vi "Hatch.vi"(10 "Polys":T4[](array[typedef]), 11 "Hatch":T4) -> (3 "Path":T2)   [LabVIEW 2014]
uses:
  TypeDefs/Poly2D.ctl
  TypeDefs/Point2D.ctl
panel:
  out "XY Graph":T3(graph)
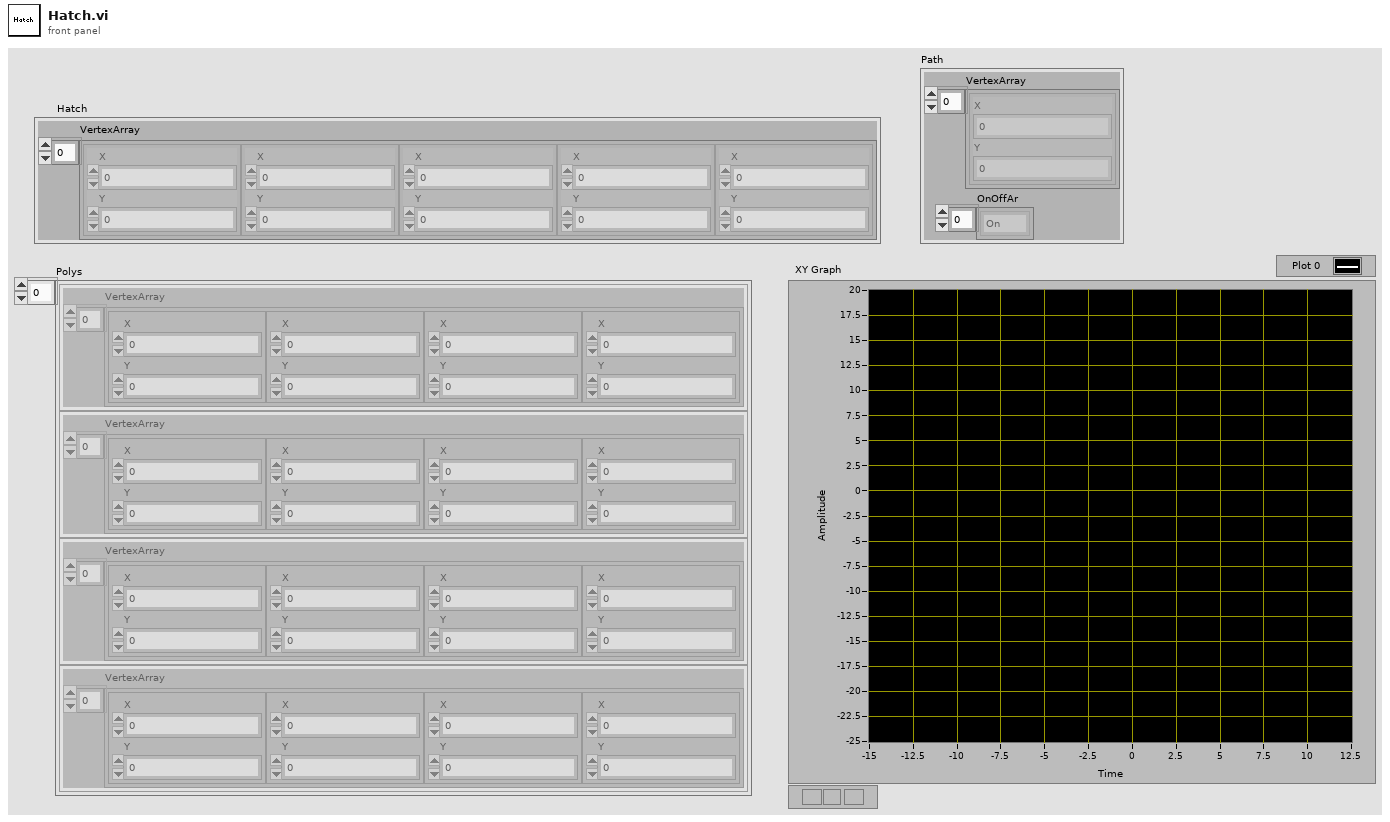
[diagram p1: front panel]
types:
  T1 = typedef "Point2D.ctl" = cluster{"X":sgl, "Y":sgl}
  T2 = cluster{"VertexArray":T1[], "OnOffAr":enum16{"On", "Off"}[]}
  T3 = cluster{"VertexArray":cluster{"X":sgl, "Y":sgl}[]}[]
  T4 = typedef "Poly2D.ctl" = cluster{"VertexArray":T1[]}
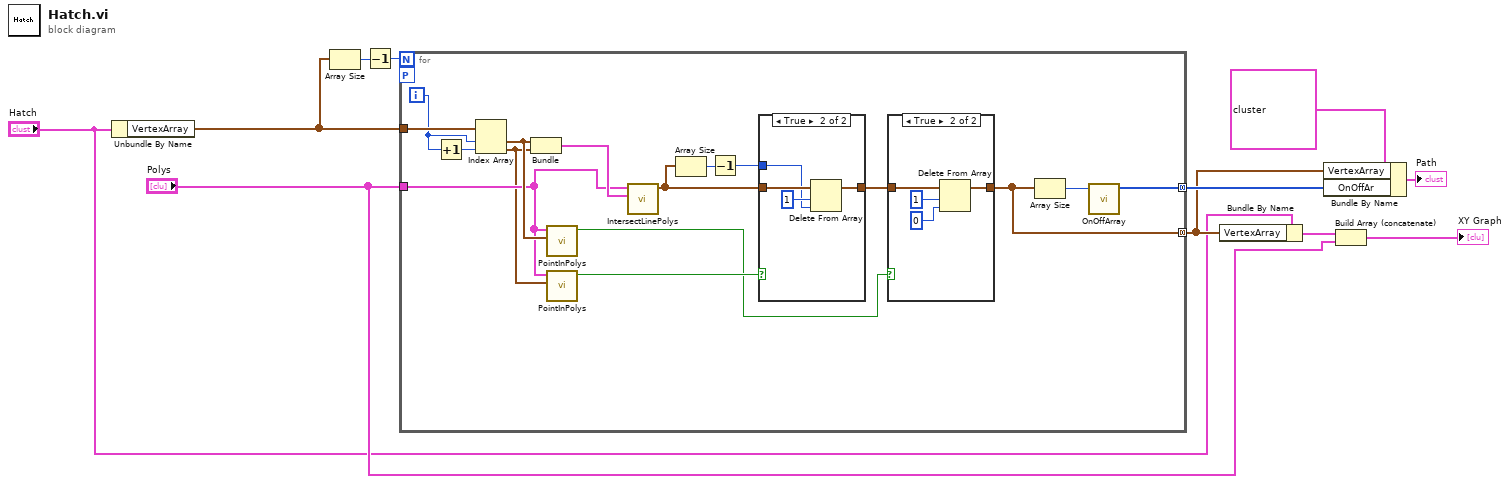
[diagram p0: block diagram]
diagram:
  n1 = Unbundle By Name("Hatch") -> ("VertexArray"=w1:T1[])
  n2 = Array Size(array=w1) -> (size(s)=w11:i32)
  n3 = Decrement(x=w11) -> (x-1=w10:i32)
  n4 = for {
    N: w10 -> [_]
    tunnel: w1 -> [w27]
    tunnel: "Polys" -> [w22]
    tunnel: [w13] -> w5 mode=concatenating
    tunnel: [w12] -> w4 mode=concatenating
    workers-P: _ -> [_]
    i -> [w25]
    n5 = Increment(x=w25) -> (x+1=w26:i32)
    n6 = Index Array(array=w27, index #1=w25, index #2=w26) -> (element #1=w24:T1, element #2=w21:T1)
    n7 = Bundle("Point2D"=w24, "Point2D"=w21) -> (w23:cluster{"Point2D":T1, "Point2D":T1})  [unwired: 1 in]
    n8 = call "PointInPolys.vi"("Point2D"=w24, "Polys"=w22) -> ("Outside"=w15:bool)  [unwired: 9 in]
    n9 = call "PointInPolys.vi"("Point2D"=w21, "Polys"=w22) -> ("Outside"=w19:bool)  [unwired: 9 in]
    n10 = call "IntersectLinePolys.vi"("Line2D"=w23, "Polys"=w22) -> ("Intersections"=w18:T1[])  [unwired: 9 in]
    n11 = Array Size(array=w18) -> (size(s)=w20:i32)
    n12 = Decrement(x=w20) -> (x-1=w17:i32)
    n13 = case shown="True" w19 {
      tunnel: w18 -> [w33 w37]
      tunnel: w17 -> [_ w35]
      tunnel: [w33 w34] -> w16
      frame False {
      }
      frame True {
        n14 = Delete From Array(array=w37, length=1, index=w35) -> (array with subset deleted=w34:T1[])  [unwired: 1 out]
      }
    }
    n15 = case shown="True" w15 {
      tunnel: w16 -> [w28 w32]
      tunnel: [w28 w30] -> w12
      frame False {
      }
      frame True {
        n16 = Delete From Array(array=w32, length=1, index=0) -> (array with subset deleted=w30:T1[])  [unwired: 1 out]
      }
    }
    n17 = Array Size(array=w12) -> (size(s)=w14:i32)
    n18 = call "OnOffArray.vi"("Size"=w14) -> ("OnOffAr"=w13:enum16{"On", "Off"}[])  [unwired: 10 in]
  }
  n19 = Bundle By Name(cluster="Hatch", "VertexArray"=w4) -> (w9:T4)
  n20 = Bundle By Name(cluster=T2 {"VertexArray"=[{"X"=-16.0, "Y"=-26.0}, {"X"=12.0, "Y"=-26.0}, {"X"=12.0, "Y"=-25.9}, {"X"=-16.0, "Y"=-25.9}, {"X"=-16.0, "Y"=-25.8}, {"X"=12.0, "Y"=-25.8}, {"X"=12.0, "Y"=-25.7}, {"X"=-16.0, "Y"=-25.7}, {"X"=-16.0, "Y"=-25.6}, {"X"=12.0, "Y"=-25.6}, {"X"=12.0, "Y"=-25.5}, {"X"=-16.0, "Y"=-25.5}, {"X"=-16.0, "Y"=-25.4}, {"X"=12.0, "Y"=-25.4}, {"X"=12.0, "Y"=-25.3}, {"X"=-16.0, "Y"=-25.3}, {"X"=-16.0, "Y"=-25.2}, {"X"=12.0, "Y"=-25.2}, {"X"=12.0, "Y"=-25.1}, {"X"=-16.0, "Y"=-25.1}, {"X"=-16.0, "Y"=-25.0}, {"X"=12.0, "Y"=-25.0}, {"X"=12.0, "Y"=-24.9}, {"X"=-16.0, "Y"=-24.9}, {"X"=-16.0, "Y"=-24.8}, {"X"=12.0, "Y"=-24.8}, {"X"=12.0, "Y"=-24.7}, {"X"=-16.0, "Y"=-24.7}, {"X"=-16.0, "Y"=-24.6}, {"X"=12.0, "Y"=-24.6}, {"X"=12.0, "Y"=-24.5}, {"X"=-16.0, "Y"=-24.5}, {"X"=-16.0, "Y"=-24.4}, {"X"=12.0, "Y"=-24.4}, {"X"=12.0, "Y"=-24.3}, {"X"=-16.0, "Y"=-24.3}, {"X"=-16.0, "Y"=-24.2}, {"X"=12.0, "Y"=-24.2}, {"X"=12.0, "Y"=-24.1}, {"X"=-16.0, "Y"=-24.1}, {"X"=-16.0, "Y"=-24.0}, {"X"=12.0, "Y"=-24.0}, {"X"=12.0, "Y"=-23.9}, {"X"=-16.0, "Y"=-23.9}, {"X"=-16.0, "Y"=-23.8}, {"X"=12.0, "Y"=-23.8}, {"X"=12.0, "Y"=-23.7}, {"X"=-16.0, "Y"=-23.7}, {"X"=-16.0, "Y"=-23.6}, {"X"=12.0, "Y"=-23.6}, {"X"=12.0, "Y"=-23.5}, {"X"=-16.0, "Y"=-23.5}, {"X"=-16.0, "Y"=-23.4}, {"X"=12.0, "Y"=-23.4}, {"X"=12.0, "Y"=-23.3}, {"X"=-16.0, "Y"=-23.3}, {"X"=-16.0, "Y"=-23.2}, {"X"=12.0, "Y"=-23.2}, {"X"=12.0, "Y"=-23.1}, {"X"=-16.0, "Y"=-23.1}, {"X"=-16.0, "Y"=-23.0}, {"X"=12.0, "Y"=-23.0}, {"X"=12.0, "Y"=-22.9}, {"X"=-16.0, "Y"=-22.9}, {"X"=-16.0, "Y"=-22.8}, {"X"=12.0, "Y"=-22.8}, {"X"=12.0, "Y"=-22.7}, {"X"=-16.0, "Y"=-22.7}, {"X"=-16.0, "Y"=-22.6}, {"X"=12.0, "Y"=-22.6}, {"X"=12.0, "Y"=-22.5}, {"X"=-16.0, "Y"=-22.5}, {"X"=-16.0, "Y"=-22.4}, {"X"=12.0, "Y"=-22.4}, {"X"=12.0, "Y"=-22.3}, {"X"=-16.0, "Y"=-22.3}, {"X"=-16.0, "Y"=-22.2}, {"X"=12.0, "Y"=-22.2}, {"X"=12.0, "Y"=-22.1}, {"X"=-16.0, "Y"=-22.1}, {"X"=-16.0, "Y"=-22.0}, {"X"=12.0, "Y"=-22.0}, {"X"=12.0, "Y"=-21.9}, {"X"=-16.0, "Y"=-21.9}, {"X"=-16.0, "Y"=-21.8}, {"X"=12.0, "Y"=-21.8}, {"X"=12.0, "Y"=-21.7}, {"X"=-16.0, "Y"=-21.7}, {"X"=-16.0, "Y"=-21.6}, {"X"=12.0, "Y"=-21.6}, {"X"=12.0, "Y"=-21.5}, {"X"=-16.0, "Y"=-21.5}, {"X"=-16.0, "Y"=-21.4}, {"X"=12.0, "Y"=-21.4}, {"X"=12.0, "Y"=-21.3}, {"X"=-16.0, "Y"=-21.3}, {"X"=-16.0, "Y"=-21.2}, {"X"=12.0, "Y"=-21.2}, {"X"=12.0, "Y"=-21.1}, {"X"=-16.0, "Y"=-21.1}, {"X"=-16.0, "Y"=-21.0}, {"X"=12.0, "Y"=-21.0}, {"X"=12.0, "Y"=-20.9}, {"X"=-16.0, "Y"=-20.9}, {"X"=-16.0, "Y"=-20.8}, {"X"=12.0, "Y"=-20.8}, {"X"=12.0, "Y"=-20.7}, {"X"=-16.0, "Y"=-20.7}, {"X"=-16.0, "Y"=-20.6}, {"X"=12.0, "Y"=-20.6}, {"X"=12.0, "Y"=-20.5}, {"X"=-16.0, "Y"=-20.5}, {"X"=-16.0, "Y"=-20.4}, {"X"=12.0, "Y"=-20.4}, {"X"=12.0, "Y"=-20.3}, {"X"=-16.0, "Y"=-20.3}, {"X"=-16.0, "Y"=-20.2}, {"X"=12.0, "Y"=-20.2}, {"X"=12.0, "Y"=-20.1}, {"X"=-16.0, "Y"=-20.1}, {"X"=-16.0, "Y"=-20.0}, {"X"=12.0, "Y"=-20.0}, {"X"=12.0, "Y"=-19.9}, {"X"=-16.0, "Y"=-19.9}, {"X"=-16.0, "Y"=-19.8}, {"X"=12.0, "Y"=-19.8}, {"X"=12.0, "Y"=-19.7}, {"X"=-16.0, "Y"=-19.7}, {"X"=-16.0, "Y"=-19.6}, {"X"=12.0, "Y"=-19.6}, {"X"=12.0, "Y"=-19.5}, {"X"=-16.0, "Y"=-19.5}, {"X"=-16.0, "Y"=-19.4}, {"X"=12.0, "Y"=-19.4}, {"X"=12.0, "Y"=-19.3}, {"X"=-16.0, "Y"=-19.3}, {"X"=-16.0, "Y"=-19.2}, {"X"=12.0, "Y"=-19.2}, {"X"=12.0, "Y"=-19.1}, {"X"=-16.0, "Y"=-19.1}, {"X"=-16.0, "Y"=-19.0}, {"X"=12.0, "Y"=-19.0}, {"X"=12.0, "Y"=-18.9}, {"X"=-16.0, "Y"=-18.9}, {"X"=-16.0, "Y"=-18.8}, {"X"=12.0, "Y"=-18.8}, {"X"=12.0, "Y"=-18.7}, {"X"=-16.0, "Y"=-18.7}, {"X"=-16.0, "Y"=-18.6}, {"X"=12.0, "Y"=-18.6}, {"X"=12.0, "Y"=-18.5}, {"X"=-16.0, "Y"=-18.5}, {"X"=-16.0, "Y"=-18.4}, {"X"=12.0, "Y"=-18.4}, {"X"=12.0, "Y"=-18.3}, {"X"=-16.0, "Y"=-18.3}, {"X"=-16.0, "Y"=-18.2}, {"X"=12.0, "Y"=-18.2}, {"X"=12.0, "Y"=-18.1}, {"X"=-16.0, "Y"=-18.1}, {"X"=-16.0, "Y"=-18.0}, {"X"=12.0, "Y"=-18.0}, {"X"=12.0, "Y"=-17.9}, {"X"=-16.0, "Y"=-17.9}, {"X"=-16.0, "Y"=-17.8}, {"X"=12.0, "Y"=-17.8}, {"X"=12.0, "Y"=-17.7}, {"X"=-16.0, "Y"=-17.7}, {"X"=-16.0, "Y"=-17.6}, {"X"=12.0, "Y"=-17.6}, {"X"=12.0, "Y"=-17.5}, {"X"=-16.0, "Y"=-17.5}, {"X"=-16.0, "Y"=-17.4}, {"X"=12.0, "Y"=-17.4}, {"X"=12.0, "Y"=-17.3}, {"X"=-16.0, "Y"=-17.3}, {"X"=-16.0, "Y"=-17.2}, {"X"=12.0, "Y"=-17.2}, {"X"=12.0, "Y"=-17.1}, {"X"=-16.0, "Y"=-17.1}, {"X"=-16.0, "Y"=-17.0}, {"X"=12.0, "Y"=-17.0}, {"X"=12.0, "Y"=-16.9}, {"X"=-16.0, "Y"=-16.9}, {"X"=-16.0, "Y"=-16.8}, {"X"=12.0, "Y"=-16.8}, {"X"=12.0, "Y"=-16.7}, {"X"=-16.0, "Y"=-16.7}, {"X"=-16.0, "Y"=-16.6}, {"X"=12.0, "Y"=-16.6}, {"X"=12.0, "Y"=-16.5}, {"X"=-16.0, "Y"=-16.5}, {"X"=-16.0, "Y"=-16.4}, {"X"=12.0, "Y"=-16.4}, {"X"=12.0, "Y"=-16.3}, {"X"=-16.0, "Y"=-16.3}, {"X"=-16.0, "Y"=-16.2}, {"X"=12.0, "Y"=-16.2}, {"X"=12.0, "Y"=-16.1}, {"X"=-16.0, "Y"=-16.1}, {"X"=-16.0, "Y"=-16.0}, {"X"=12.0, "Y"=-16.0}, {"X"=12.0, "Y"=-15.9}, {"X"=-16.0, "Y"=-15.9}, {"X"=-16.0, "Y"=-15.8}, {"X"=12.0, "Y"=-15.8}, {"X"=12.0, "Y"=-15.7}, {"X"=-16.0, "Y"=-15.7}, {"X"=-16.0, "Y"=-15.6}, {"X"=12.0, "Y"=-15.6}, {"X"=12.0, "Y"=-15.5}, {"X"=-16.0, "Y"=-15.5}, {"X"=-16.0, "Y"=-15.4}, {"X"=12.0, "Y"=-15.4}, {"X"=12.0, "Y"=-15.3}, {"X"=-16.0, "Y"=-15.3}, {"X"=-16.0, "Y"=-15.2}, {"X"=12.0, "Y"=-15.2}, {"X"=12.0, "Y"=-15.1}, {"X"=-16.0, "Y"=-15.1}, {"X"=-16.0, "Y"=-15.0}, {"X"=12.0, "Y"=-15.0}, {"X"=12.0, "Y"=-14.9}, {"X"=-16.0, "Y"=-14.9}, {"X"=-16.0, "Y"=-14.8}, {"X"=12.0, "Y"=-14.8}, {"X"=12.0, "Y"=-14.7}, {"X"=-16.0, "Y"=-14.7}, {"X"=-16.0, "Y"=-14.6}, {"X"=12.0, "Y"=-14.6}, {"X"=12.0, "Y"=-14.5}, {"X"=-16.0, "Y"=-14.5}, {"X"=-16.0, "Y"=-14.4}, {"X"=12.0, "Y"=-14.4}, {"X"=12.0, "Y"=-14.3}, {"X"=-16.0, "Y"=-14.3}, {"X"=-16.0, "Y"=-14.2}, {"X"=12.0, "Y"=-14.2}, {"X"=12.0, "Y"=-14.1}, {"X"=-16.0, "Y"=-14.1}, {"X"=-16.0, "Y"=-14.0}, {"X"=12.0, "Y"=-14.0}, {"X"=12.0, "Y"=-13.9}, {"X"=-16.0, "Y"=-13.9}, {"X"=-16.0, "Y"=-13.8}, {"X"=12.0, "Y"=-13.8}, {"X"=12.0, "Y"=-13.7}, {"X"=-16.0, "Y"=-13.7}, {"X"=-16.0, "Y"=-13.6}, {"X"=12.0, "Y"=-13.6}, {"X"=12.0, "Y"=-13.5}, {"X"=-16.0, "Y"=-13.5}, {"X"=-16.0, "Y"=-13.4}, {"X"=12.0, "Y"=-13.4}, {"X"=12.0, "Y"=-13.3}, {"X"=-16.0, "Y"=-13.3}, {"X"=-16.0, "Y"=-13.2}, {"X"=12.0, "Y"=-13.2}, {"X"=12.0, "Y"=-13.1}, {"X"=-16.0, "Y"=-13.1}, {"X"=-16.0, "Y"=-13.0}, {"X"=12.0, "Y"=-13.0}, {"X"=12.0, "Y"=-12.9}, {"X"=-16.0, "Y"=-12.9}, {"X"=-16.0, "Y"=-12.8}, {"X"=12.0, "Y"=-12.8}, {"X"=12.0, "Y"=-12.7}, {"X"=-16.0, "Y"=-12.7}, {"X"=-16.0, "Y"=-12.6}, {"X"=12.0, "Y"=-12.6}, {"X"=12.0, "Y"=-12.5}, {"X"=-16.0, "Y"=-12.5}, {"X"=-16.0, "Y"=-12.4}, {"X"=12.0, "Y"=-12.4}, {"X"=12.0, "Y"=-12.3}, {"X"=-16.0, "Y"=-12.3}, {"X"=-16.0, "Y"=-12.2}, {"X"=12.0, "Y"=-12.2}, {"X"=12.0, "Y"=-12.1}, {"X"=-16.0, "Y"=-12.1}, {"X"=-16.0, "Y"=-12.0}, {"X"=12.0, "Y"=-12.0}, {"X"=12.0, "Y"=-11.9}, {"X"=-16.0, "Y"=-11.9}, {"X"=-16.0, "Y"=-11.8}, {"X"=12.0, "Y"=-11.8}, {"X"=12.0, "Y"=-11.7}, {"X"=-16.0, "Y"=-11.7}, {"X"=-16.0, "Y"=-11.6}, {"X"=12.0, "Y"=-11.6}, {"X"=12.0, "Y"=-11.5}, {"X"=-16.0, "Y"=-11.5}, {"X"=-16.0, "Y"=-11.4}, {"X"=12.0, "Y"=-11.4}, {"X"=12.0, "Y"=-11.3}, {"X"=-16.0, "Y"=-11.3}, {"X"=-16.0, "Y"=-11.2}, {"X"=12.0, "Y"=-11.2}, {"X"=12.0, "Y"=-11.1}, {"X"=-16.0, "Y"=-11.1}, {"X"=-16.0, "Y"=-11.0}, {"X"=12.0, "Y"=-11.0}, {"X"=12.0, "Y"=-10.9}, {"X"=-16.0, "Y"=-10.9}, {"X"=-16.0, "Y"=-10.8}, {"X"=12.0, "Y"=-10.8}, {"X"=12.0, "Y"=-10.7}, {"X"=-16.0, "Y"=-10.7}, {"X"=-16.0, "Y"=-10.6}, {"X"=12.0, "Y"=-10.6}, {"X"=12.0, "Y"=-10.5}, {"X"=-16.0, "Y"=-10.5}, {"X"=-16.0, "Y"=-10.4}, {"X"=12.0, "Y"=-10.4}, {"X"=12.0, "Y"=-10.3}, {"X"=-16.0, "Y"=-10.3}, {"X"=-16.0, "Y"=-10.2}, {"X"=12.0, "Y"=-10.2}, {"X"=12.0, "Y"=-10.1}, {"X"=-16.0, "Y"=-10.1}, {"X"=-16.0, "Y"=-10.0}, {"X"=12.0, "Y"=-10.0}, {"X"=12.0, "Y"=-9.9}, {"X"=-16.0, "Y"=-9.9}, {"X"=-16.0, "Y"=-9.8}, {"X"=12.0, "Y"=-9.8}, {"X"=12.0, "Y"=-9.7}, {"X"=-16.0, "Y"=-9.7}, {"X"=-16.0, "Y"=-9.6}, {"X"=12.0, "Y"=-9.6}, {"X"=12.0, "Y"=-9.5}, {"X"=-16.0, "Y"=-9.5}, {"X"=-16.0, "Y"=-9.4}, {"X"=12.0, "Y"=-9.4}, {"X"=12.0, "Y"=-9.3}, {"X"=-16.0, "Y"=-9.3}, {"X"=-16.0, "Y"=-9.2}, {"X"=12.0, "Y"=-9.2}, {"X"=12.0, "Y"=-9.1}, {"X"=-16.0, "Y"=-9.1}, {"X"=-16.0, "Y"=-9.0}, {"X"=12.0, "Y"=-9.0}, {"X"=12.0, "Y"=-8.9}, {"X"=-16.0, "Y"=-8.9}, {"X"=-16.0, "Y"=-8.8}, {"X"=12.0, "Y"=-8.8}, {"X"=12.0, "Y"=-8.7}, {"X"=-16.0, "Y"=-8.7}, {"X"=-16.0, "Y"=-8.6}, {"X"=12.0, "Y"=-8.6}, {"X"=12.0, "Y"=-8.5}, {"X"=-16.0, "Y"=-8.5}, {"X"=-16.0, "Y"=-8.4}, {"X"=12.0, "Y"=-8.4}, {"X"=12.0, "Y"=-8.3}, {"X"=-16.0, "Y"=-8.3}, {"X"=-16.0, "Y"=-8.2}, {"X"=12.0, "Y"=-8.2}, {"X"=12.0, "Y"=-8.1}, {"X"=-16.0, "Y"=-8.1}, {"X"=-16.0, "Y"=-8.0}, {"X"=12.0, "Y"=-8.0}, {"X"=12.0, "Y"=-7.9}, {"X"=-16.0, "Y"=-7.9}, {"X"=-16.0, "Y"=-7.8}, {"X"=12.0, "Y"=-7.8}, {"X"=12.0, "Y"=-7.7}, {"X"=-16.0, "Y"=-7.7}, {"X"=-16.0, "Y"=-7.6}, {"X"=12.0, "Y"=-7.6}, {"X"=12.0, "Y"=-7.5}, {"X"=-16.0, "Y"=-7.5}, {"X"=-16.0, "Y"=-7.4}, {"X"=12.0, "Y"=-7.4}, {"X"=12.0, "Y"=-7.3}, {"X"=-16.0, "Y"=-7.3}, {"X"=-16.0, "Y"=-7.2}, {"X"=12.0, "Y"=-7.2}, {"X"=12.0, "Y"=-7.1}, {"X"=-16.0, "Y"=-7.1}, {"X"=-16.0, "Y"=-7.0}, {"X"=12.0, "Y"=-7.0}, {"X"=12.0, "Y"=-6.9}, {"X"=-16.0, "Y"=-6.9}, {"X"=-16.0, "Y"=-6.8}, {"X"=12.0, "Y"=-6.8}, {"X"=12.0, "Y"=-6.7}, {"X"=-16.0, "Y"=-6.7}, {"X"=-16.0, "Y"=-6.6}, {"X"=12.0, "Y"=-6.6}, {"X"=12.0, "Y"=-6.5}, {"X"=-16.0, "Y"=-6.5}, {"X"=-16.0, "Y"=-6.4}, {"X"=12.0, "Y"=-6.4}, {"X"=12.0, "Y"=-6.3}, {"X"=-16.0, "Y"=-6.3}, {"X"=-16.0, "Y"=-6.2}, {"X"=12.0, "Y"=-6.2}, {"X"=12.0, "Y"=-6.1}, {"X"=-16.0, "Y"=-6.1}, {"X"=-16.0, "Y"=-6.0}, {"X"=12.0, "Y"=-6.0}, {"X"=12.0, "Y"=-5.9}, {"X"=-16.0, "Y"=-5.9}, {"X"=-16.0, "Y"=-5.8}, {"X"=12.0, "Y"=-5.8}, {"X"=12.0, "Y"=-5.7}, {"X"=-16.0, "Y"=-5.7}, {"X"=-16.0, "Y"=-5.6}, {"X"=12.0, "Y"=-5.6}, {"X"=12.0, "Y"=-5.5}, {"X"=-16.0, "Y"=-5.5}, {"X"=-16.0, "Y"=-5.4}, {"X"=12.0, "Y"=-5.4}, {"X"=12.0, "Y"=-5.3}, {"X"=-16.0, "Y"=-5.3}, {"X"=-16.0, "Y"=-5.2}, {"X"=12.0, "Y"=-5.2}, {"X"=12.0, "Y"=-5.1}, {"X"=-16.0, "Y"=-5.1}, {"X"=-16.0, "Y"=-5.0}, {"X"=12.0, "Y"=-5.0}, {"X"=12.0, "Y"=-4.9}, {"X"=-16.0, "Y"=-4.9}, {"X"=-16.0, "Y"=-4.8}, {"X"=12.0, "Y"=-4.8}, {"X"=12.0, "Y"=-4.7}, {"X"=-16.0, "Y"=-4.7}, {"X"=-16.0, "Y"=-4.6}, {"X"=12.0, "Y"=-4.6}, {"X"=12.0, "Y"=-4.5}, {"X"=-16.0, "Y"=-4.5}, {"X"=-16.0, "Y"=-4.4}, {"X"=12.0, "Y"=-4.4}, {"X"=12.0, "Y"=-4.3}, {"X"=-16.0, "Y"=-4.3}, {"X"=-16.0, "Y"=-4.2}, {"X"=12.0, "Y"=-4.2}, {"X"=12.0, "Y"=-4.1}, {"X"=-16.0, "Y"=-4.1}, {"X"=-16.0, "Y"=-4.0}, {"X"=12.0, "Y"=-4.0}, {"X"=12.0, "Y"=-3.9}, {"X"=-16.0, "Y"=-3.9}, {"X"=-16.0, "Y"=-3.8}, {"X"=12.0, "Y"=-3.8}, {"X"=12.0, "Y"=-3.7}, {"X"=-16.0, "Y"=-3.7}, {"X"=-16.0, "Y"=-3.6}, {"X"=12.0, "Y"=-3.6}, {"X"=12.0, "Y"=-3.5}, {"X"=-16.0, "Y"=-3.5}, {"X"=-16.0, "Y"=-3.4}, {"X"=12.0, "Y"=-3.4}, {"X"=12.0, "Y"=-3.3}, {"X"=-16.0, "Y"=-3.3}, {"X"=-16.0, "Y"=-3.2}, {"X"=12.0, "Y"=-3.2}, {"X"=12.0, "Y"=-3.1}, {"X"=-16.0, "Y"=-3.1}, {"X"=-16.0, "Y"=-3.0}, {"X"=12.0, "Y"=-3.0}, {"X"=12.0, "Y"=-2.9}, {"X"=-16.0, "Y"=-2.9}, {"X"=-16.0, "Y"=-2.8}, {"X"=12.0, "Y"=-2.8}, {"X"=12.0, "Y"=-2.7}, {"X"=-16.0, "Y"=-2.7}, {"X"=-16.0, "Y"=-2.6}, {"X"=12.0, "Y"=-2.6}, {"X"=12.0, "Y"=-2.5}, {"X"=-16.0, "Y"=-2.5}, {"X"=-16.0, "Y"=-2.4}, {"X"=12.0, "Y"=-2.4}, {"X"=12.0, "Y"=-2.3}, {"X"=-16.0, "Y"=-2.3}, {"X"=-16.0, "Y"=-2.2}, {"X"=12.0, "Y"=-2.2}, {"X"=12.0, "Y"=-2.1}, {"X"=-16.0, "Y"=-2.1}, {"X"=-16.0, "Y"=-2.0}, {"X"=12.0, "Y"=-2.0}, {"X"=12.0, "Y"=-1.9}, {"X"=-16.0, "Y"=-1.9}, {"X"=-16.0, "Y"=-1.8}, {"X"=12.0, "Y"=-1.8}, {"X"=12.0, "Y"=-1.7}, {"X"=-16.0, "Y"=-1.7}, {"X"=-16.0, "Y"=-1.6}, {"X"=12.0, "Y"=-1.6}, {"X"=12.0, "Y"=-1.5}, {"X"=-16.0, "Y"=-1.5}, {"X"=-16.0, "Y"=-1.4}, {"X"=12.0, "Y"=-1.4}, {"X"=12.0, "Y"=-1.3}, {"X"=-16.0, "Y"=-1.3}, {"X"=-16.0, "Y"=-1.2}, {"X"=12.0, "Y"=-1.2}, {"X"=12.0, "Y"=-1.1}, {"X"=-16.0, "Y"=-1.1}, {"X"=-16.0, "Y"=-1.0}, {"X"=12.0, "Y"=-1.0}, {"X"=12.0, "Y"=-0.9}, {"X"=-16.0, "Y"=-0.9}, {"X"=-16.0, "Y"=-0.8}, {"X"=12.0, "Y"=-0.8}, {"X"=12.0, "Y"=-0.7}, {"X"=-16.0, "Y"=-0.7}, {"X"=-16.0, "Y"=-0.6}, {"X"=12.0, "Y"=-0.6}, {"X"=12.0, "Y"=-0.5}, {"X"=-16.0, "Y"=-0.5}, {"X"=-16.0, "Y"=-0.4}, {"X"=12.0, "Y"=-0.4}, {"X"=12.0, "Y"=-0.3}, {"X"=-16.0, "Y"=-0.3}, {"X"=-16.0, "Y"=-0.2}, {"X"=12.0, "Y"=-0.2}, {"X"=12.0, "Y"=-0.1}, {"X"=-16.0, "Y"=-0.1}, {"X"=-16.0, "Y"=0.0}, {"X"=12.0, "Y"=0.0}, {"X"=12.0, "Y"=0.1}, {"X"=-16.0, "Y"=0.1}, {"X"=-16.0, "Y"=0.2}, {"X"=12.0, "Y"=0.2}, {"X"=12.0, "Y"=0.3}, {"X"=-16.0, "Y"=0.3}, {"X"=-16.0, "Y"=0.4}, {"X"=12.0, "Y"=0.4}, {"X"=12.0, "Y"=0.5}, {"X"=-16.0, "Y"=0.5}, {"X"=-16.0, "Y"=0.6}, {"X"=12.0, "Y"=0.6}, {"X"=12.0, "Y"=0.7}, {"X"=-16.0, "Y"=0.7}, {"X"=-16.0, "Y"=0.8}, {"X"=12.0, "Y"=0.8}, {"X"=12.0, "Y"=0.9}, {"X"=-16.0, "Y"=0.9}, {"X"=-16.0, "Y"=1.0}, {"X"=12.0, "Y"=1.0}, {"X"=12.0, "Y"=1.1}, {"X"=-16.0, "Y"=1.1}, {"X"=-16.0, "Y"=1.2}, {"X"=12.0, "Y"=1.2}, {"X"=12.0, "Y"=1.3}, {"X"=-16.0, "Y"=1.3}, {"X"=-16.0, "Y"=1.4}, {"X"=12.0, "Y"=1.4}, {"X"=12.0, "Y"=1.5}, {"X"=-16.0, "Y"=1.5}, {"X"=-16.0, "Y"=1.6}, {"X"=12.0, "Y"=1.6}, {"X"=12.0, "Y"=1.7}, {"X"=-16.0, "Y"=1.7}, {"X"=-16.0, "Y"=1.8}, {"X"=12.0, "Y"=1.8}, {"X"=12.0, "Y"=1.9}, {"X"=-16.0, "Y"=1.9}, {"X"=-16.0, "Y"=2.0}, {"X"=12.0, "Y"=2.0}, {"X"=12.0, "Y"=2.1}, {"X"=-16.0, "Y"=2.1}, {"X"=-16.0, "Y"=2.2}, {"X"=12.0, "Y"=2.2}, {"X"=12.0, "Y"=2.3}, {"X"=-16.0, "Y"=2.3}, {"X"=-16.0, "Y"=2.4}, {"X"=12.0, "Y"=2.4}, {"X"=12.0, "Y"=2.5}, {"X"=-16.0, "Y"=2.5}, {"X"=-16.0, "Y"=2.6}, {"X"=12.0, "Y"=2.6}, {"X"=12.0, "Y"=2.7}, {"X"=-16.0, "Y"=2.7}, {"X"=-16.0, "Y"=2.8}, {"X"=12.0, "Y"=2.8}, {"X"=12.0, "Y"=2.9}, {"X"=-16.0, "Y"=2.9}, {"X"=-16.0, "Y"=3.0}, {"X"=12.0, "Y"=3.0}, {"X"=12.0, "Y"=3.1}, {"X"=-16.0, "Y"=3.1}, {"X"=-16.0, "Y"=3.2}, {"X"=12.0, "Y"=3.2}, {"X"=12.0, "Y"=3.3}, {"X"=-16.0, "Y"=3.3}, {"X"=-16.0, "Y"=3.4}, {"X"=12.0, "Y"=3.4}, {"X"=12.0, "Y"=3.5}, {"X"=-16.0, "Y"=3.5}, {"X"=-16.0, "Y"=3.6}, {"X"=12.0, "Y"=3.6}, {"X"=12.0, "Y"=3.7}, {"X"=-16.0, "Y"=3.7}, {"X"=-16.0, "Y"=3.8}, {"X"=12.0, "Y"=3.8}, {"X"=12.0, "Y"=3.9}, {"X"=-16.0, "Y"=3.9}, {"X"=-16.0, "Y"=4.0}, {"X"=12.0, "Y"=4.0}, {"X"=12.0, "Y"=4.1}, {"X"=-16.0, "Y"=4.1}, {"X"=-16.0, "Y"=4.2}, {"X"=12.0, "Y"=4.2}, {"X"=12.0, "Y"=4.3}, {"X"=-16.0, "Y"=4.3}, {"X"=-16.0, "Y"=4.4}, {"X"=12.0, "Y"=4.4}, {"X"=12.0, "Y"=4.5}, {"X"=-16.0, "Y"=4.5}, {"X"=-16.0, "Y"=4.6}, {"X"=12.0, "Y"=4.6}, {"X"=12.0, "Y"=4.7}, {"X"=-16.0, "Y"=4.7}, {"X"=-16.0, "Y"=4.8}, {"X"=12.0, "Y"=4.8}, {"X"=12.0, "Y"=4.9}, {"X"=-16.0, "Y"=4.9}, {"X"=-16.0, "Y"=5.0}, {"X"=12.0, "Y"=5.0}, {"X"=12.0, "Y"=5.1}, {"X"=-16.0, "Y"=5.1}, {"X"=-16.0, "Y"=5.2}, {"X"=12.0, "Y"=5.2}, {"X"=12.0, "Y"=5.3}, {"X"=-16.0, "Y"=5.3}, {"X"=-16.0, "Y"=5.4}, {"X"=12.0, "Y"=5.4}, {"X"=12.0, "Y"=5.5}, {"X"=-16.0, "Y"=5.5}, {"X"=-16.0, "Y"=5.6}, {"X"=12.0, "Y"=5.6}, {"X"=12.0, "Y"=5.7}, {"X"=-16.0, "Y"=5.7}, {"X"=-16.0, "Y"=5.8}, {"X"=12.0, "Y"=5.8}, {"X"=12.0, "Y"=5.9}, {"X"=-16.0, "Y"=5.9}, {"X"=-16.0, "Y"=6.0}, {"X"=12.0, "Y"=6.0}, {"X"=12.0, "Y"=6.1}, {"X"=-16.0, "Y"=6.1}, {"X"=-16.0, "Y"=6.2}, {"X"=12.0, "Y"=6.2}, {"X"=12.0, "Y"=6.3}, {"X"=-16.0, "Y"=6.3}, {"X"=-16.0, "Y"=6.4}, {"X"=12.0, "Y"=6.4}, {"X"=12.0, "Y"=6.5}, {"X"=-16.0, "Y"=6.5}, {"X"=-16.0, "Y"=6.6}, {"X"=12.0, "Y"=6.6}, {"X"=12.0, "Y"=6.7}, {"X"=-16.0, "Y"=6.7}, {"X"=-16.0, "Y"=6.8}, {"X"=12.0, "Y"=6.8}, {"X"=12.0, "Y"=6.9}, {"X"=-16.0, "Y"=6.9}, {"X"=-16.0, "Y"=7.0}, {"X"=12.0, "Y"=7.0}, {"X"=12.0, "Y"=7.1}, {"X"=-16.0, "Y"=7.1}, {"X"=-16.0, "Y"=7.2}, {"X"=12.0, "Y"=7.2}, {"X"=12.0, "Y"=7.3}, {"X"=-16.0, "Y"=7.3}, {"X"=-16.0, "Y"=7.4}, {"X"=12.0, "Y"=7.4}, {"X"=12.0, "Y"=7.5}, {"X"=-16.0, "Y"=7.5}, {"X"=-16.0, "Y"=7.6}, {"X"=12.0, "Y"=7.6}, {"X"=12.0, "Y"=7.7}, {"X"=-16.0, "Y"=7.7}, {"X"=-16.0, "Y"=7.8}, {"X"=12.0, "Y"=7.8}, {"X"=12.0, "Y"=7.9}, {"X"=-16.0, "Y"=7.9}, {"X"=-16.0, "Y"=8.0}, {"X"=12.0, "Y"=8.0}, {"X"=12.0, "Y"=8.1}, {"X"=-16.0, "Y"=8.1}, {"X"=-16.0, "Y"=8.2}, {"X"=12.0, "Y"=8.2}, {"X"=12.0, "Y"=8.3}, {"X"=-16.0, "Y"=8.3}, {"X"=-16.0, "Y"=8.4}, {"X"=12.0, "Y"=8.4}, {"X"=12.0, "Y"=8.5}, {"X"=-16.0, "Y"=8.5}, {"X"=-16.0, "Y"=8.6}, {"X"=12.0, "Y"=8.6}, {"X"=12.0, "Y"=8.7}, {"X"=-16.0, "Y"=8.7}, {"X"=-16.0, "Y"=8.8}, {"X"=12.0, "Y"=8.8}, {"X"=12.0, "Y"=8.9}, {"X"=-16.0, "Y"=8.9}, {"X"=-16.0, "Y"=9.0}, {"X"=12.0, "Y"=9.0}, {"X"=12.0, "Y"=9.1}, {"X"=-16.0, "Y"=9.1}, {"X"=-16.0, "Y"=9.2}, {"X"=12.0, "Y"=9.2}, {"X"=12.0, "Y"=9.3}, {"X"=-16.0, "Y"=9.3}, {"X"=-16.0, "Y"=9.4}, {"X"=12.0, "Y"=9.4}, {"X"=12.0, "Y"=9.5}, {"X"=-16.0, "Y"=9.5}, {"X"=-16.0, "Y"=9.6}, {"X"=12.0, "Y"=9.6}, {"X"=12.0, "Y"=9.7}, {"X"=-16.0, "Y"=9.7}, {"X"=-16.0, "Y"=9.8}, {"X"=12.0, "Y"=9.8}, {"X"=12.0, "Y"=9.9}, {"X"=-16.0, "Y"=9.9}, {"X"=-16.0, "Y"=10.0}, {"X"=12.0, "Y"=10.0}, {"X"=12.0, "Y"=10.1}, {"X"=-16.0, "Y"=10.1}, {"X"=-16.0, "Y"=10.2}, {"X"=12.0, "Y"=10.2}, {"X"=12.0, "Y"=10.3}, {"X"=-16.0, "Y"=10.3}, {"X"=-16.0, "Y"=10.4}, {"X"=12.0, "Y"=10.4}, {"X"=12.0, "Y"=10.5}, {"X"=-16.0, "Y"=10.5}, {"X"=-16.0, "Y"=10.6}, {"X"=12.0, "Y"=10.6}, {"X"=12.0, "Y"=10.7}, {"X"=-16.0, "Y"=10.7}, {"X"=-16.0, "Y"=10.8}, {"X"=12.0, "Y"=10.8}, {"X"=12.0, "Y"=10.9}, {"X"=-16.0, "Y"=10.9}, {"X"=-16.0, "Y"=11.0}, {"X"=12.0, "Y"=11.0}, {"X"=12.0, "Y"=11.1}, {"X"=-16.0, "Y"=11.1}, {"X"=-16.0, "Y"=11.2}, {"X"=12.0, "Y"=11.2}, {"X"=12.0, "Y"=11.3}, {"X"=-16.0, "Y"=11.3}, {"X"=-16.0, "Y"=11.4}, {"X"=12.0, "Y"=11.4}, {"X"=12.0, "Y"=11.5}, {"X"=-16.0, "Y"=11.5}, {"X"=-16.0, "Y"=11.6}, {"X"=12.0, "Y"=11.6}, {"X"=12.0, "Y"=11.7}, {"X"=-16.0, "Y"=11.7}, {"X"=-16.0, "Y"=11.8}, {"X"=12.0, "Y"=11.8}, {"X"=12.0, "Y"=11.9}, {"X"=-16.0, "Y"=11.9}, {"X"=-16.0, "Y"=12.0}, {"X"=12.0, "Y"=12.0}, {"X"=12.0, "Y"=12.1}, {"X"=-16.0, "Y"=12.1}, {"X"=-16.0, "Y"=12.2}, {"X"=12.0, "Y"=12.2}, {"X"=12.0, "Y"=12.3}, {"X"=-16.0, "Y"=12.3}, {"X"=-16.0, "Y"=12.4}, {"X"=12.0, "Y"=12.4}, {"X"=12.0, "Y"=12.5}, {"X"=-16.0, "Y"=12.5}, {"X"=-16.0, "Y"=12.6}, {"X"=12.0, "Y"=12.6}, {"X"=12.0, "Y"=12.7}, {"X"=-16.0, "Y"=12.7}, {"X"=-16.0, "Y"=12.8}, {"X"=12.0, "Y"=12.8}, {"X"=12.0, "Y"=12.9}, {"X"=-16.0, "Y"=12.9}, {"X"=-16.0, "Y"=13.0}, {"X"=12.0, "Y"=13.0}, {"X"=12.0, "Y"=13.1}, {"X"=-16.0, "Y"=13.1}, {"X"=-16.0, "Y"=13.2}, {"X"=12.0, "Y"=13.2}, {"X"=12.0, "Y"=13.3}, {"X"=-16.0, "Y"=13.3}, {"X"=-16.0, "Y"=13.4}, {"X"=12.0, "Y"=13.4}, {"X"=12.0, "Y"=13.5}, {"X"=-16.0, "Y"=13.5}, {"X"=-16.0, "Y"=13.6}, {"X"=12.0, "Y"=13.6}, {"X"=12.0, "Y"=13.7}, {"X"=-16.0, "Y"=13.7}, {"X"=-16.0, "Y"=13.8}, {"X"=12.0, "Y"=13.8}, {"X"=12.0, "Y"=13.9}, {"X"=-16.0, "Y"=13.9}, {"X"=-16.0, "Y"=14.0}, {"X"=12.0, "Y"=14.0}, {"X"=12.0, "Y"=14.1}, {"X"=-16.0, "Y"=14.1}, {"X"=-16.0, "Y"=14.2}, {"X"=12.0, "Y"=14.2}, {"X"=12.0, "Y"=14.3}, {"X"=-16.0, "Y"=14.3}, {"X"=-16.0, "Y"=14.4}, {"X"=12.0, "Y"=14.4}, {"X"=12.0, "Y"=14.5}, {"X"=-16.0, "Y"=14.5}, {"X"=-16.0, "Y"=14.6}, {"X"=12.0, "Y"=14.6}, {"X"=12.0, "Y"=14.7}, {"X"=-16.0, "Y"=14.7}, {"X"=-16.0, "Y"=14.8}, {"X"=12.0, "Y"=14.8}, {"X"=12.0, "Y"=14.9}, {"X"=-16.0, "Y"=14.9}, {"X"=-16.0, "Y"=15.0}, {"X"=12.0, "Y"=15.0}, {"X"=12.0, "Y"=15.1}, {"X"=-16.0, "Y"=15.1}, {"X"=-16.0, "Y"=15.2}, {"X"=12.0, "Y"=15.2}, {"X"=12.0, "Y"=15.3}, {"X"=-16.0, "Y"=15.3}, {"X"=-16.0, "Y"=15.4}, {"X"=12.0, "Y"=15.4}, {"X"=12.0, "Y"=15.5}, {"X"=-16.0, "Y"=15.5}, {"X"=-16.0, "Y"=15.6}, {"X"=12.0, "Y"=15.6}, {"X"=12.0, "Y"=15.7}, {"X"=-16.0, "Y"=15.7}, {"X"=-16.0, "Y"=15.8}, {"X"=12.0, "Y"=15.8}, {"X"=12.0, "Y"=15.9}, {"X"=-16.0, "Y"=15.9}, {"X"=-16.0, "Y"=16.0}, {"X"=12.0, "Y"=16.0}, {"X"=12.0, "Y"=16.1}, {"X"=-16.0, "Y"=16.1}, {"X"=-16.0, "Y"=16.2}, {"X"=12.0, "Y"=16.2}, {"X"=12.0, "Y"=16.3}, {"X"=-16.0, "Y"=16.3}, {"X"=-16.0, "Y"=16.4}, {"X"=12.0, "Y"=16.4}, {"X"=12.0, "Y"=16.5}, {"X"=-16.0, "Y"=16.5}, {"X"=-16.0, "Y"=16.6}, {"X"=12.0, "Y"=16.6}, {"X"=12.0, "Y"=16.7}, {"X"=-16.0, "Y"=16.7}, {"X"=-16.0, "Y"=16.8}, {"X"=12.0, "Y"=16.8}, {"X"=12.0, "Y"=16.9}, {"X"=-16.0, "Y"=16.9}, {"X"=-16.0, "Y"=17.0}, {"X"=12.0, "Y"=17.0}, {"X"=12.0, "Y"=17.1}, {"X"=-16.0, "Y"=17.1}, {"X"=-16.0, "Y"=17.2}, {"X"=12.0, "Y"=17.2}, {"X"=12.0, "Y"=17.3}, {"X"=-16.0, "Y"=17.3}, {"X"=-16.0, "Y"=17.4}, {"X"=12.0, "Y"=17.4}, {"X"=12.0, "Y"=17.5}, {"X"=-16.0, "Y"=17.5}, {"X"=-16.0, "Y"=17.6}, {"X"=12.0, "Y"=17.6}, {"X"=12.0, "Y"=17.7}, {"X"=-16.0, "Y"=17.7}, {"X"=-16.0, "Y"=17.8}, {"X"=12.0, "Y"=17.8}, {"X"=12.0, "Y"=17.9}, {"X"=-16.0, "Y"=17.9}, {"X"=-16.0, "Y"=18.0}, {"X"=12.0, "Y"=18.0}, {"X"=12.0, "Y"=18.1}, {"X"=-16.0, "Y"=18.1}, {"X"=-16.0, "Y"=18.2}, {"X"=12.0, "Y"=18.2}, {"X"=12.0, "Y"=18.3}, {"X"=-16.0, "Y"=18.3}, {"X"=-16.0, "Y"=18.4}, {"X"=12.0, "Y"=18.4}, {"X"=12.0, "Y"=18.5}, {"X"=-16.0, "Y"=18.5}, {"X"=-16.0, "Y"=18.6}, {"X"=12.0, "Y"=18.6}, {"X"=12.0, "Y"=18.7}, {"X"=-16.0, "Y"=18.7}, {"X"=-16.0, "Y"=18.8}, {"X"=12.0, "Y"=18.8}, {"X"=12.0, "Y"=18.9}, {"X"=-16.0, "Y"=18.9}, {"X"=-16.0, "Y"=19.0}, {"X"=12.0, "Y"=19.0}, {"X"=12.0, "Y"=19.1}, {"X"=-16.0, "Y"=19.1}, {"X"=-16.0, "Y"=19.2}, {"X"=12.0, "Y"=19.2}, {"X"=12.0, "Y"=19.3}, {"X"=-16.0, "Y"=19.3}, {"X"=-16.0, "Y"=19.4}, {"X"=12.0, "Y"=19.4}, {"X"=12.0, "Y"=19.5}, {"X"=-16.0, "Y"=19.5}, {"X"=-16.0, "Y"=19.6}, {"X"=12.0, "Y"=19.6}, {"X"=12.0, "Y"=19.7}, {"X"=-16.0, "Y"=19.7}, {"X"=-16.0, "Y"=19.8}, {"X"=12.0, "Y"=19.8}, {"X"=12.0, "Y"=19.9}, {"X"=-16.0, "Y"=19.9}], "OnOffAr"=[]} ("Poly2D"), "VertexArray"=w4, "OnOffAr"=w5) -> (→"Path":T2)
  n21 = Build Array (concatenate)(w9, "Polys") -> (→"XY Graph":T4[])
